vi "GetLeftSR.vi"(8 "error in":errorcluster, 11 "RightShiftRegister in":refnum<class "RightShiftRegister.lvclass">) -> (0 "error out":errorcluster, 3 "RightShiftRegister out":refnum<class "RightShiftRegister.lvclass">, 5 "left SR":i32[](array[numeric]))   [LabVIEW 2014, in "RightShiftRegister.lvclass"]
uses:
  RightShiftRegister.lvclass
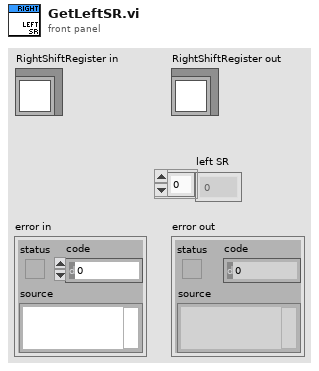
[diagram p1: front panel]
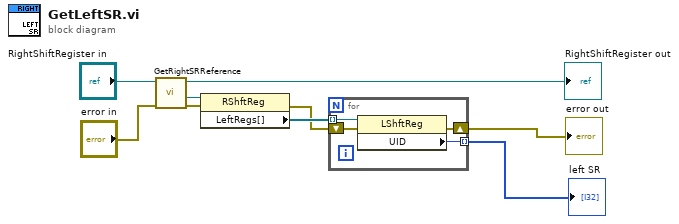
[diagram p0: block diagram]
diagram:
  n1 = call "GetRightSRReference.vi"("error in"="error in", "ShiftRegister in"="RightShiftRegister in") -> ("error out"=w6:errorcluster, "reference out"=w7:refnum<vi>, "ShiftRegister out"=→"RightShiftRegister out":refnum<class "RightShiftRegister.lvclass">)  [unwired: 7 in]
  n2 = property class="RShftReg"(reference=w7, error in=w6) -> (error out=w4:errorcluster, "LeftRegs[]"=w5:refnum<vi>[])  [unwired: 1 out]
  n3 = for {
    tunnel: w5 -> [w12] mode=indexing
    shift-right: [w11] -> w3
    shift-left: w4 -> [w13]
    tunnel: [w10] -> w1 mode=indexing
    n4 = property class="LShftReg"(reference=w12, error in=w13) -> (error out=w11:errorcluster, "UID"=w10:i32)  [unwired: 1 out]
  }
  "error out" <- w3
  "left SR" <- w1
